vi "OpenConnection_Control2.vi"(8 "error in (no error)":errorcluster, 9 "type":T1, 10 "topicName":string) -> (0 "error out":errorcluster, 3 "reference":refnum<vi>)   [LabVIEW 2012]
uses:
  Typedefs/Control 2.ctl
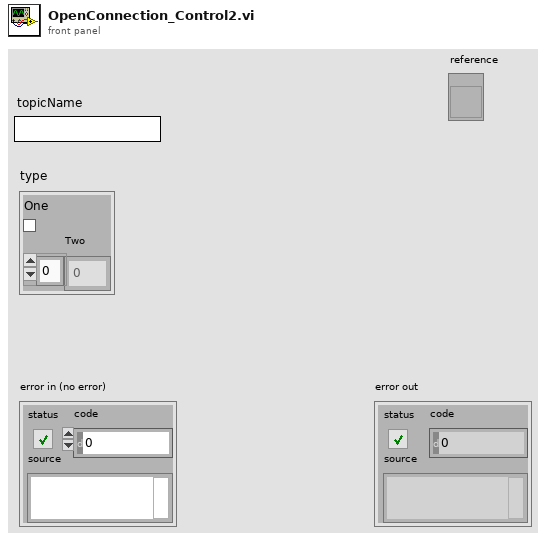
[diagram p1: front panel]
types:
  T1 = typedef "Control 2.ctl" = cluster{"One":bool, "Two":i32[]}
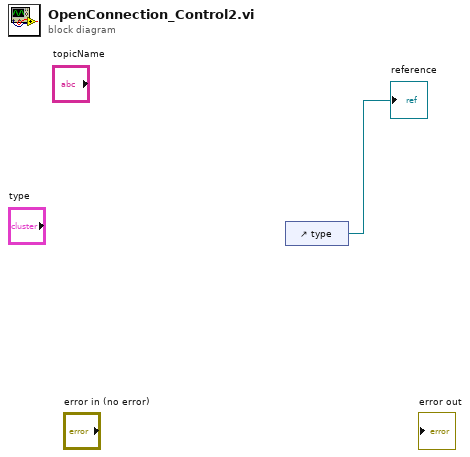
[diagram p0: block diagram]
diagram:
  n1 = control-ref of="type"() -> (→"reference":refnum<vi>)
